vi "confirm active and inactive modules.vi"() -> ()   [LabVIEW 2012]
doc: "SciScan 1.2 160622"
panel:
  in  "inactive modules IN":string[](array[string])
  in  "optional modules IN":string[](array[string])
  in  "required modules IN":string[](array[string])
  in  "stop":bool
  in  "inactive modules":i32(listbox)
  in  "optional modules":i32(listbox)
  in  "required modules":i32(listbox)
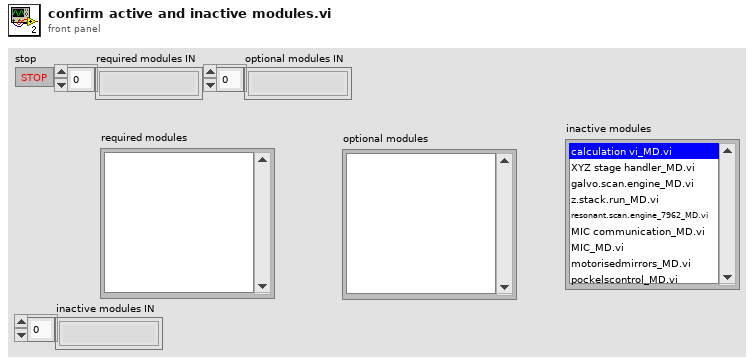
[diagram p1: front panel]
types:
  T1 = cluster{"data name":string, "drag data":variant}[]
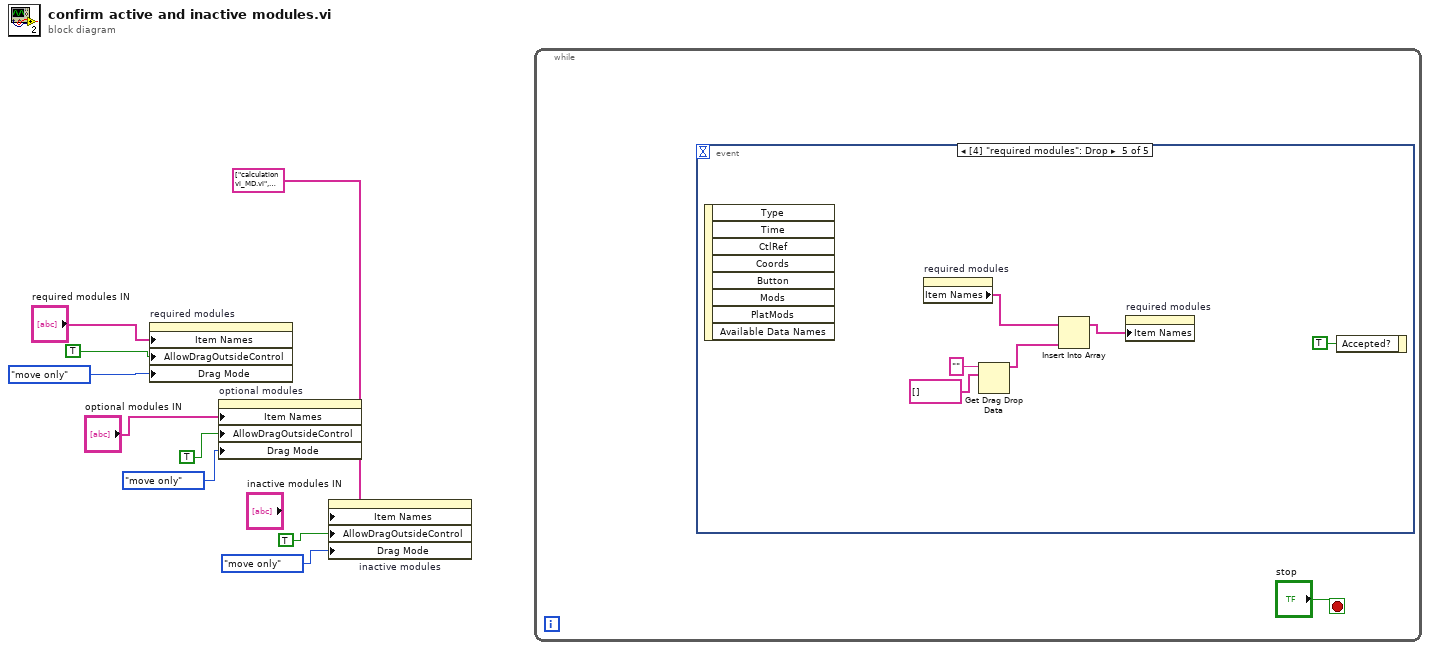
[diagram p0: block diagram]
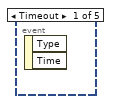
[diagram p2: hidden frame]
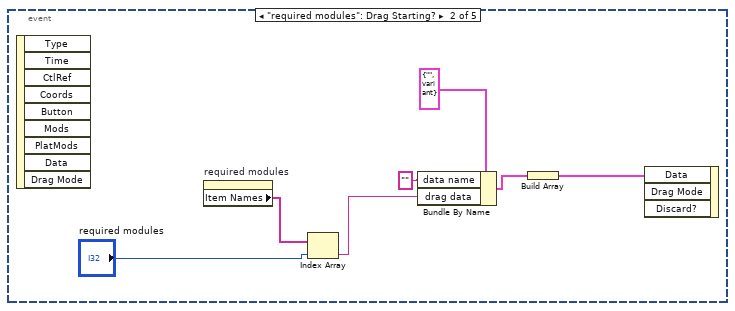
[diagram p3: hidden frame]
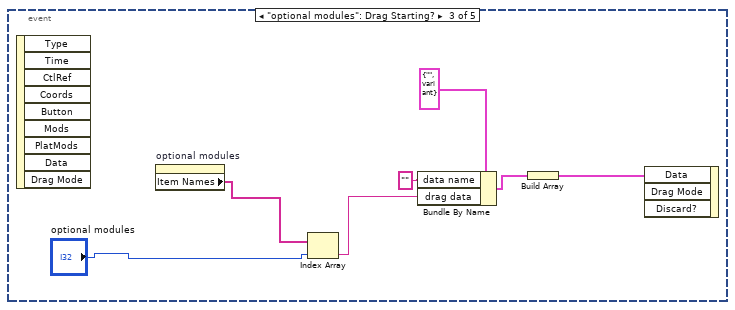
[diagram p4: hidden frame]
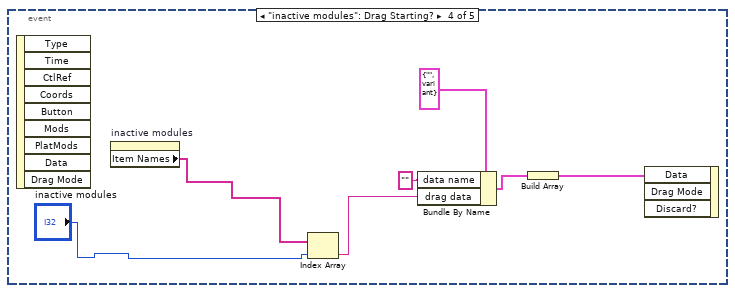
[diagram p5: hidden frame]
diagram:
  n1 = property on="required modules" class="LstBox (strict)"("Item Names"="required modules IN", "AllowDragOutsideControl"=TRUE ("Drag/Drop:Allow Drag and Drop Outside Control"), "Drag Mode"=enum32{"copy or move", "copy only", "move only"}."move only" ("Drag/Drop:Drag Mode")) -> ()  [unwired: 2 in, 2 out]
  n2 = property on="optional modules" class="LstBox (strict)"("Item Names"="optional modules IN", "AllowDragOutsideControl"=TRUE ("Drag/Drop:Allow Drag and Drop Outside Control"), "Drag Mode"=enum32{"copy or move", "copy only", "move only"}."move only" ("Drag/Drop:Drag Mode")) -> ()  [unwired: 2 in, 2 out]
  n3 = property on="inactive modules" class="LstBox (strict)"("Item Names"=string[] ["calculation vi_MD.vi", "XYZ stage handler_MD.vi", "galvo.scan.engine_MD.vi", "z.stack.run_MD.vi", "resonant.scan.engine_7962_MD.vi", "MIC communication_MD.vi", "MIC_MD.vi", "motorisedmirrors_MD.vi", "pockelscontrol_MD.vi", "pockelscontrol_w_blanking_for_PXI6259_MD.vi", "MOCK XYZ stage communication_MD.vi", "display queue to fp display_MD.vi", "image queue to disk and to display queue_MD.vi", "raw queue to image queue_MD.vi", "load_external_coordinates_MD.vi", "make arbitrary waveform_MD.vi", "standard frame scan geometry_MD.vi", "MacroLoopManager_MD.vi", "MacroOpsManager_MD.vi", "MacroStagePositioning_MD.vi", "Initialize_MacroGUI_MD.vi", "MacroGUI_MD.vi"] ("inactive modules"), "AllowDragOutsideControl"=TRUE ("Drag/Drop:Allow Drag and Drop Outside Control"), "Drag Mode"=enum32{"copy or move", "copy only", "move only"}."move only" ("Drag/Drop:Drag Mode")) -> ()  [unwired: 2 in, 2 out]
  n4 = while {
    stop <- "stop" stop-if-true
    n5 = event shown="[4] \"required modules\": Drop" {
      selector: _ -> [_ _ _ _ _]
      dyn-events: _ -> [_ _ _ _ _]
      timeout: _ -> [_ _ _ _ _]
      event Timeout {
        n6 = event-data() -> ()  [unwired: 1 in, 2 out]
      }
      event "required modules": Drag Starting? {
        n7 = event-data() -> ()  [unwired: 1 in, 9 out]
        n8 = property on="required modules" class="LstBox (strict)"() -> ("Item Names"=w17:string[])  [unwired: 2 in, 2 out]
        n9 = Index Array(array=w17, index="required modules") -> (element=w13:string)
        n10 = Bundle By Name(cluster=cluster{"data name":string, "drag data":variant} {"data name"="", "drag data"=variant}, "data name"="", "drag data"=w13) -> (w12:cluster{"data name":string, "drag data":variant})
        n11 = Build Array(w12) -> (w11:T1)
        n12 = event-data("Data"=w11) -> ()  [unwired: 3 in, 1 out]
      }
      event "optional modules": Drag Starting? {
        n13 = event-data() -> ()  [unwired: 1 in, 9 out]
        n14 = property on="optional modules" class="LstBox (strict)"() -> ("Item Names"=w18:string[])  [unwired: 2 in, 2 out]
        n15 = Index Array(array=w18, index="optional modules") -> (element=w22:string)
        n16 = Bundle By Name(cluster=cluster{"data name":string, "drag data":variant} {"data name"="", "drag data"=variant}, "data name"="", "drag data"=w22) -> (w21:cluster{"data name":string, "drag data":variant})
        n17 = Build Array(w21) -> (w20:T1)
        n18 = event-data("Data"=w20) -> ()  [unwired: 3 in, 1 out]
      }
      event "inactive modules": Drag Starting? {
        n19 = event-data() -> ()  [unwired: 1 in, 9 out]
        n20 = property on="inactive modules" class="LstBox (strict)"() -> ("Item Names"=w25:string[])  [unwired: 2 in, 2 out]
        n21 = Index Array(array=w25, index="inactive modules") -> (element=w29:string)
        n22 = Bundle By Name(cluster=cluster{"data name":string, "drag data":variant} {"data name"="", "drag data"=variant}, "data name"="", "drag data"=w29) -> (w28:cluster{"data name":string, "drag data":variant})
        n23 = Build Array(w28) -> (w27:T1)
        n24 = event-data("Data"=w27) -> ()  [unwired: 3 in, 1 out]
      }
      event "required modules": Drop {
        n25 = event-data() -> ()  [unwired: 1 in, 8 out]
        n26 = property on="required modules" class="LstBox (strict)"() -> ("Item Names"=w33:string[])  [unwired: 2 in, 2 out]
        n27 = Get Drag Drop Data(8:string[] [] ("subarray"), 9:"" ("data name")) -> (3:w34:string[])  [unwired: 1 in, 1 out]
        n28 = Insert Into Array(array=w33, new element=w34) -> (w32:string[])  [unwired: 1 in]
        n29 = property on="required modules" class="LstBox (strict)"("Item Names"=w32) -> ()  [unwired: 2 in, 2 out]
        n30 = event-data("Accepted?"=TRUE) -> ()  [unwired: 1 in, 1 out]
      }
    }
  }
